vi "SaveData_WL.vi"(3 "Data W-L":T1, 4 "Name":string(combo)="WL_UP_", 5 "Lane_Number":string(combo)="ST1_") -> (2 "new file path":path)   [LabVIEW 2017]
uses:
  <vilib>/Utility/file.llb/Read Delimited Spreadsheet (string).vi
  <vilib>/Utility/file.llb/Write Delimited Spreadsheet (string).vi
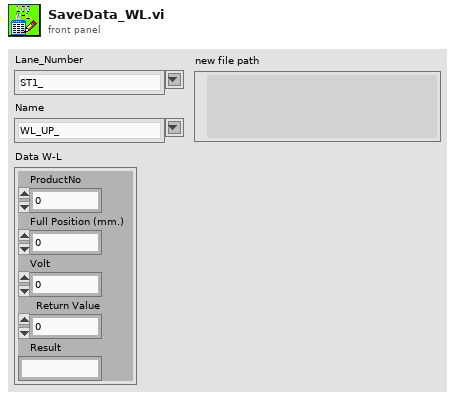
[diagram p1: front panel]
types:
  T1 = cluster{"ProductNo":u16, "Full Position (mm.)":dbl, "Volt":dbl, "Return Value":dbl, "Result":string}
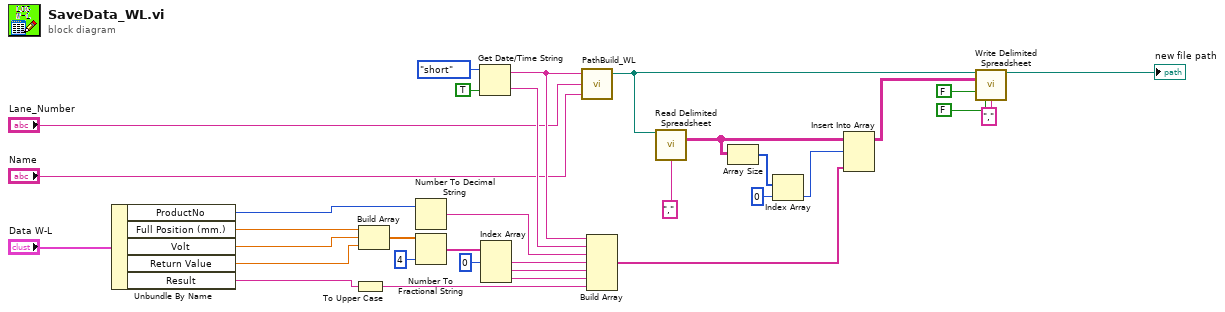
[diagram p0: block diagram]
diagram:
  n1 = Unbundle By Name("Data W-L") -> ("ProductNo"=w7:u16, "Full Position (mm.)"=w15:dbl, "Volt"=w6:dbl, "Return Value"=w14:dbl, "Result"=w5:string)
  n2 = To Upper Case(1:w5) -> (0:w4:string)
  n3 = Build Array(w15, w6, w14) -> (w31:dbl[])
  n4 = Number To Decimal String(number=w7) -> (decimal integer string=w12:string)  [unwired: 1 in]
  n5 = Number To Fractional String(number=w31, precision (6)=i16 4) -> (F-format string=w29:string[])  [unwired: 2 in]
  n6 = Get Date/Time String(date format (0)=enum16{"short", "long", "abbreviated"}."short", want seconds? (F)=TRUE) -> (date string=w32:string, time string=w27:string)  [unwired: 1 in]
  n7 = Index Array(array=w29, index #1=0 ("index")) -> (element #1=w11:string, element #2=w10:string, element #3=w9:string)  [unwired: 2 in]
  n8 = call "PathBuild_WL.vi"("Name"="Name", "Lane_Number"="Lane_Number", "Date"=w32) -> ("path"=w23:path)  [unwired: 2 in]
  n9 = Build Array "Build Array"(w32, w27, w12, w11, w10, w9, w4) -> (w33:string[])
  n10 = call-poly <vilib>:"Read Delimited Spreadsheet.vi"("file path (dialog if empty)"=w23, "delimiter (\\t)"="," ("delimiter (\\t)")) -> ("all rows"=w21:string[][])  [unwired: 8 in, 5 out]
  n11 = Array Size(array=w21) -> (size(s)=w20:i32[])
  n12 = Index Array(array=w20, index=0) -> (element=w18:i32)
  n13 = Insert Into Array "Insert Into Array"(array=w21, index (row)=w18, new element=w33) -> (w24:string[][])  [unwired: 1 in]
  n14 = call-poly <vilib>:"Write Delimited Spreadsheet.vi"("file path (dialog if empty)"=w23, "2D data"=w24, "append to file? (new file:F)"=FALSE, "transpose? (no:F)"=FALSE, "delimiter (\\t)"="," ("delimiter (\\t)")) -> ("new file path (Not A Path if cancelled)"=→"new file path":path)  [unwired: 9 in, 1 out]
